vi "CameraAction.vi"(8 "FrontTarget":bool, 9 "BackDown":bool, 10 "FrontLevel":bool, 11 "BackLevel":bool) -> ()   [LabVIEW 2015]
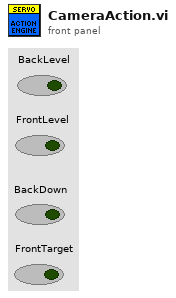
[diagram p1: front panel]
types:
  T1 = typedef "WPI_ServoDeviceRef.ctl" = cluster{"DeviceStatus":errorcluster, "PWM Channel":T2, "DeadBand":T3}
  T2 = typedef "FPGA_DIOPWMChannel.ctl" = enum8{"PWM 0", "PWM 1", "PWM 2", "PWM 3", "PWM 4", "PWM 5", "PWM 6", "PWM 7", "PWM 8", "PWM 9", "PWM MXP 0", "PWM MXP 1", "PWM MXP 2", "PWM MXP 3", "PWM MXP 4", "PWM MXP 5", "PWM MXP 6", "PWM MXP 7", "PWM MXP 8", "PWM MXP 9", "Invalid"}
  T3 = typedef "WPI_PWMDeadband.ctl" = cluster{"Name":string, "maxPositivePwm":i32, "minPositivePwm":i32, "centerPwm":i32, "maxNegativePwm":i32, "minNegativePwm":i32, "angularRange":u16}
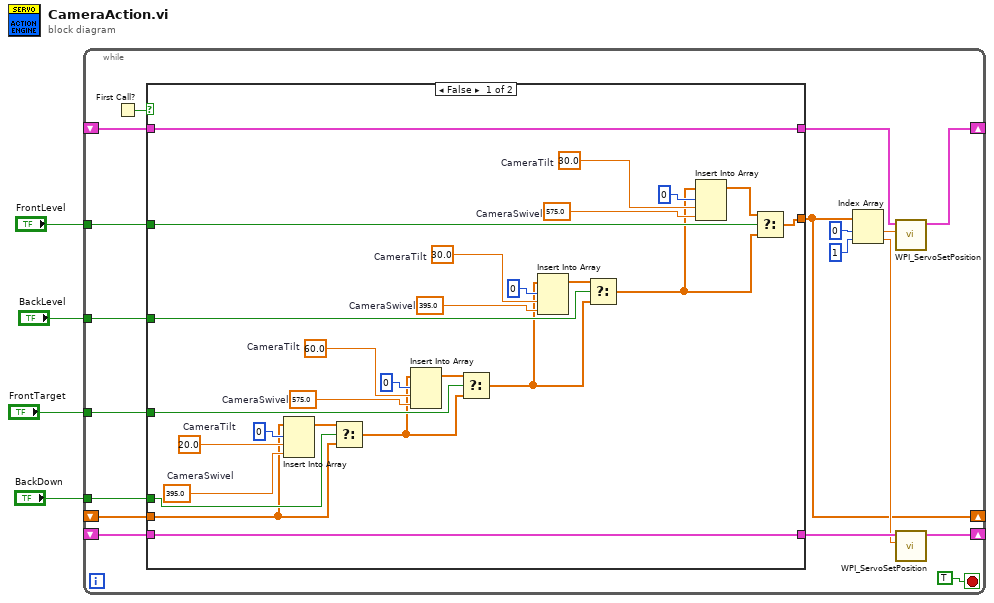
[diagram p0: block diagram]
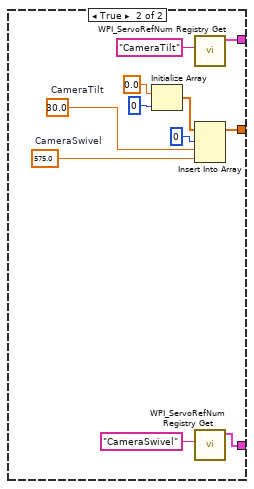
[diagram p2: hidden frame]
diagram:
  n1 = while {
    tunnel: "BackLevel" -> [w21]
    tunnel: "FrontLevel" -> [w20]
    tunnel: "BackDown" -> [w19]
    tunnel: "FrontTarget" -> [w18]
    shift-right: [w15] -> _
    shift-left: _ -> [w11]
    shift-right: [w13] -> _
    shift-left: _ -> [w12]
    shift-right: [w6] -> _
    shift-left: _ -> [w5]
    stop <- TRUE stop-if-true
    n2 = First Call?() -> (First Call?: T/F=w17:bool)
    n3 = case shown="False" w17 {
      tunnel: w21 -> [w49 _]
      tunnel: w20 -> [w48 _]
      tunnel: w19 -> [w47 _]
      tunnel: w18 -> [w46 _]
      tunnel: [w44 w58] -> w16
      tunnel: [w45 w57] -> w14
      tunnel: w12 -> [w45 _]
      tunnel: w11 -> [w44 _]
      tunnel: [w43 w50] -> w6
      tunnel: w5 -> [w24 _]
      frame False {
        w33 = 575.0  # CameraSwivel
        w32 = 30.0  # CameraTilt
        w34 = 395.0  # CameraSwivel
        w35 = 30.0  # CameraTilt
        w39 = 395.0  # CameraSwivel
        w38 = 20.0  # CameraTilt
        w42 = 575.0  # CameraSwivel
        w41 = 60.0  # CameraTilt
        n4 = Insert Into Array(array=w24, index=0, new element #1=w38, new element #2=w39) -> (w28:dbl[])
        n5 = Select(t=w28, s=w47, f=w24) -> (s? t:f=w23:dbl[])
        n6 = Insert Into Array(array=w23, index=0, new element #1=w41, new element #2=w42) -> (w27:dbl[])
        n7 = Select(t=w27, s=w46, f=w23) -> (s? t:f=w25:dbl[])
        n8 = Insert Into Array(array=w25, index=0, new element #1=w35, new element #2=w34) -> (w30:dbl[])
        n9 = Select(t=w30, s=w49, f=w25) -> (s? t:f=w26:dbl[])
        n10 = Insert Into Array(array=w26, index=0, new element #1=w32, new element #2=w33) -> (w29:dbl[])
        n11 = Select(t=w29, s=w48, f=w26) -> (s? t:f=w43:dbl[])
      }
      frame True {
        w52 = 575.0  # CameraSwivel
        w53 = 30.0  # CameraTilt
        n12 = Initialize Array(0.0 ("element"), 0 ("dimension size")) -> (w54:dbl[])
        n13 = call <vilib>:"WPI_ServoRefNum Registry Get.vi"("refnum name"="CameraTilt") -> ("ServoDeviceRef"=w58:T1)  [unwired: 9 in, 1 out]
        n14 = Insert Into Array(array=w54, index=0, new element #1=w53, new element #2=w52) -> (w50:dbl[])
        n15 = call <vilib>:"WPI_ServoRefNum Registry Get.vi"("refnum name"="CameraSwivel") -> ("ServoDeviceRef"=w57:T1)  [unwired: 9 in, 1 out]
      }
    }
    n16 = Index Array(array=w6, index #1=0 ("index"), index #2=1 ("index")) -> (element #1=w8:dbl, element #2=w7:dbl)
    n17 = call <vilib>:"WPI_ServoSetPosition.vi"("Position"=w8, "ServoDeviceRef"=w16) -> ("ServoDeviceRef"=w15:T1)  [unwired: 8 in, 1 out]
    n18 = call <vilib>:"WPI_ServoSetPosition.vi"("Position"=w7, "ServoDeviceRef"=w14) -> ("ServoDeviceRef"=w13:T1)  [unwired: 8 in, 1 out]
  }
